vi "Actor Core.vi"(8 "error in":errorcluster, 11 "FirstAF in":refnum<class "FirstAF.lvclass">) -> (0 "error out":errorcluster, 3 "Actor out":refnum<class "Actor.lvclass">)   [LabVIEW 2019, in "FirstAF.lvlib" / "FirstAF.lvclass"]
doc: "(<B>Filename</B>: Actor Framework.lvlib:Actor.lvclass:Actor Core.vi)\n\nReceives messages to the actor, reacts to them, and initiates any error handling that may shut the actor down.\n\nDescendant classes may override this VI to append parallel tasks for the actor to complete while it handles messages. Overrides use the Call Parent Method node."
uses:
  FirstAF.lvclass
  C:/Program Files (x86)/National Instruments/LabVIEW 2019/vi.lib/ActorFramework/Actor/Actor.lvclass
  <vilib>/ActorFramework/Actor/Actor.lvclass
  <vilib>/ActorFramework/Actor/Actor.lvclass/Actor.ctl
  <vilib>/ActorFramework/Message Enqueuer/Message Enqueuer.lvclass/Message Enqueuer.ctl
  FirstAF.lvclass/FirstAF.ctl
  FirstAF Messages/Increment Msg/Increment Msg.lvclass/Increment Msg.ctl
  FirstAF Messages/Decrement Msg/Decrement Msg.lvclass/Decrement Msg.ctl
  <vilib>/ActorFramework/Message Enqueuer/Init from Existing Queue.vi
  <vilib>/ActorFramework/Message Enqueuer/Enqueue.vi
  FirstAF Messages/Increment Msg/Increment Msg.lvclass
  C:/Program Files (x86)/National Instruments/LabVIEW 2019/vi.lib/ActorFramework/Message/Message.lvclass
  <vilib>/ActorFramework/Stop Msg/Stop Msg.lvclass
  FirstAF Messages/Decrement Msg/Decrement Msg.lvclass
  <vilib>/ActorFramework/Message Priority Queue/Priority Enqueue.vi
  <vilib>/ActorFramework/Message Enqueuer/Message Enqueuer.lvclass
panel:
  out "Result":i32
  in  "Stop":bool
  in  "Amount":i32
  in  "Decrement":bool
  in  "Increment":bool
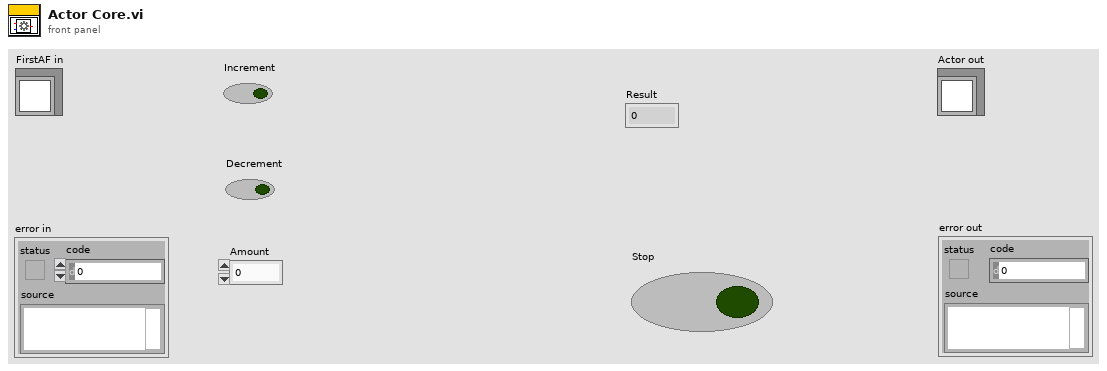
[diagram p1: front panel]
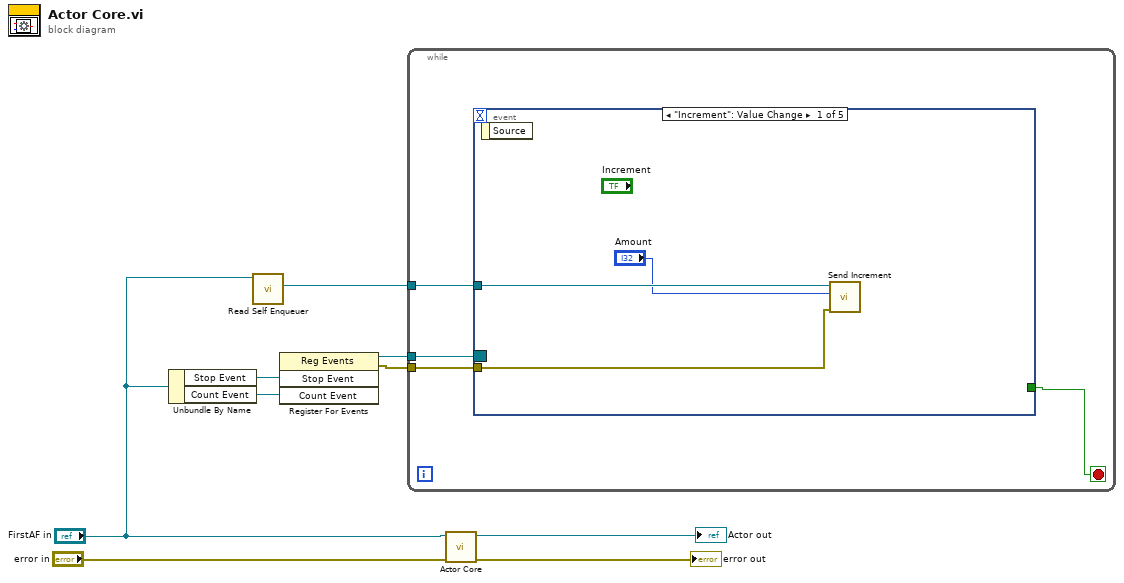
[diagram p0: block diagram]
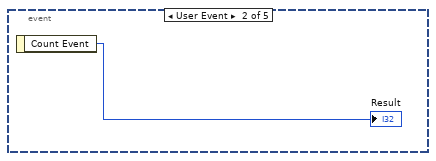
[diagram p2: hidden frame]
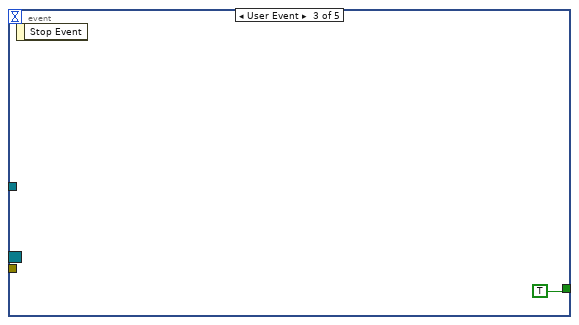
[diagram p3: hidden frame]
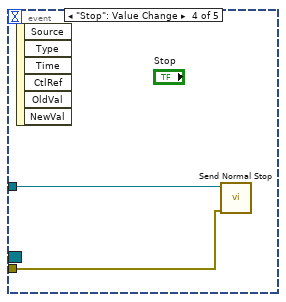
[diagram p4: hidden frame]
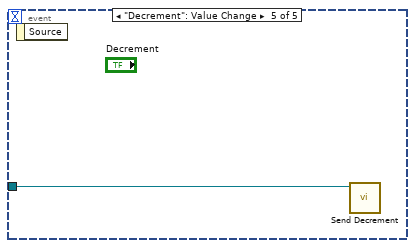
[diagram p5: hidden frame]
diagram:
  n1 = Unbundle By Name("FirstAF in") -> ("Stop Event"=w2:refnum<user-event>, "Count Event"=w1:refnum<user-event>)
  n2 = call <vilib>:"Read Self Enqueuer.vi"("Actor"="FirstAF in") -> ("Self Enqueuer"=w4:refnum<class "Message Enqueuer.lvclass">)  [unwired: 10 in]
  n3 = register-events(w2, w1) -> (reference out=w6:refnum<event-registration>, error out=w3:errorcluster)  [unwired: 2 in]
  n4 = while {
    tunnel: w6 -> [w13]
    tunnel: w4 -> [w12]
    tunnel: w3 -> [w11]
    stop <- w10 stop-if-true
    n5 = event shown="[0] \"Increment\": Value Change" {
      selector: w13 -> [_ _ _ _ _]
      dyn-events: _ -> [_ _ _ _ _]
      timeout: _ -> [_ _ _ _ _]
      tunnel: w12 -> [w16 _ _ w20 w21]
      tunnel: w11 -> [w14 _ _ w19 _]
      tunnel: [_ _ TRUE _ _] -> w10
      event "Increment": Value Change {
        n6 = event-data() -> ()  [unwired: 1 in, 1 out]
        n7 = call "Send Increment.vi"("error in (no error)"=w14, "Amount"="Amount", "Message Enqueuer"=w16) -> ()  [unwired: 7 in, 2 out]
      }
      event User Event {
        n8 = event-data() -> ("Count Event"=→"Result":i32)  [unwired: 1 in]
      }
      event User Event {
        n9 = event-data() -> ()  [unwired: 1 in, 1 out]
      }
      event "Stop": Value Change {
        n10 = event-data() -> ()  [unwired: 1 in, 6 out]
        n11 = call <vilib>:"Send Normal Stop.vi"("error in (no error)"=w19, "Message Enqueuer"=w20) -> ()  [unwired: 9 in, 1 out]
      }
      event "Decrement": Value Change {
        n12 = event-data() -> ()  [unwired: 1 in, 1 out]
        n13 = call "Send Decrement.vi"("Message Enqueuer"=w21) -> ()  [unwired: 9 in, 2 out]
      }
    }
  }
  n14 = call-parent "Actor Core.vi"("error in"="error in", "Actor in"="FirstAF in") -> ("error out"=→"error out":errorcluster, "Actor out"=→"Actor out":refnum<class "Actor.lvclass">)  [unwired: 8 in]
